vi "GetLibPath.vi"(8 "error in (no error)":errorcluster) -> (0 "error out":errorcluster, 3 "Path":path)   [LabVIEW 2020, in "CameraI2COUSB.lvlib" / "CameraI2COUSB.lvclass"]
uses:
  CameraI2COUSB.lvclass
  CameraI2COUSB.lvclass/CameraI2COUSB.ctl
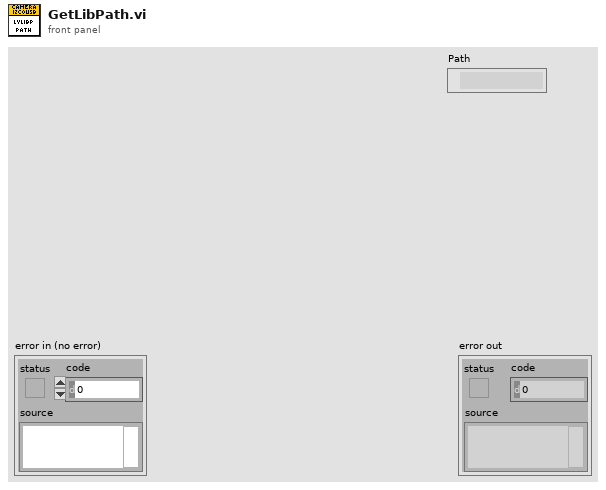
[diagram p1: front panel]
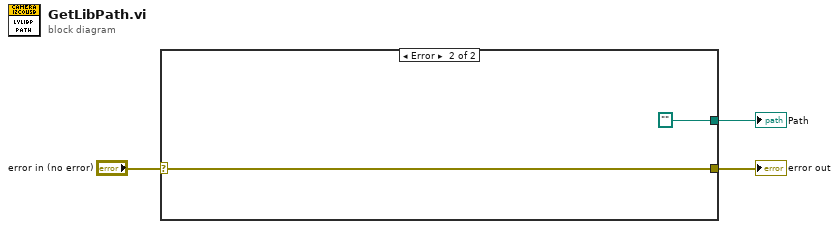
[diagram p0: block diagram]
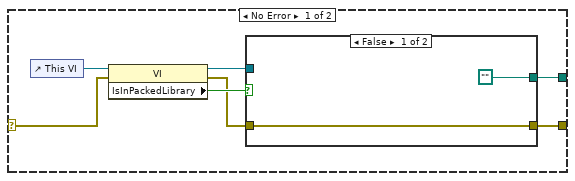
[diagram p2: hidden frame]
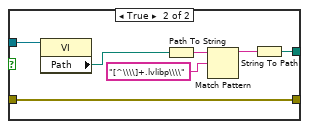
[diagram p3: hidden frame]
diagram:
  n1 = case shown="Error" "error in (no error)" {
    selector: "error in (no error)" -> [w10 w21]
    tunnel: [w6 w21] -> w2
    tunnel: [w4 path ""] -> w1
    frame No Error {
      n2 = control-ref of="This VI"() -> (w5:refnum<vi>)
      n3 = property class="VI"(reference=w5, error in=w10) -> (reference out=w7:refnum<vi>, error out=w8:errorcluster, "IsInPackedLibrary"=w9:bool)
      n4 = case shown="False" w9 {
        tunnel: w8 -> [w12 w14]
        tunnel: w7 -> [_ w16]
        tunnel: [w12 w14] -> w6
        tunnel: [path "" w13] -> w4
        frame False {
        }
        frame True {
          n5 = property class="VI"(reference=w16) -> ("Path"=w15:path)  [unwired: 1 in, 2 out]
          n6 = Path To String(path=w15) -> (string=w19:string)
          n7 = Match Pattern(string=w19, regular expression="[^\\\\]+.lvlibp\\\\") -> (before substring=w17:string)  [unwired: 1 in, 3 out]
          n8 = String To Path(string=w17) -> (path=w13:path)
        }
      }
    }
    frame Error {
    }
  }
  "error out" <- w2
  "Path" <- w1
